vi "udp_test.vi"() -> ()   [LabVIEW 2013]
panel:
  out "data out":string
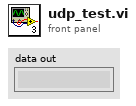
[diagram p1: front panel]
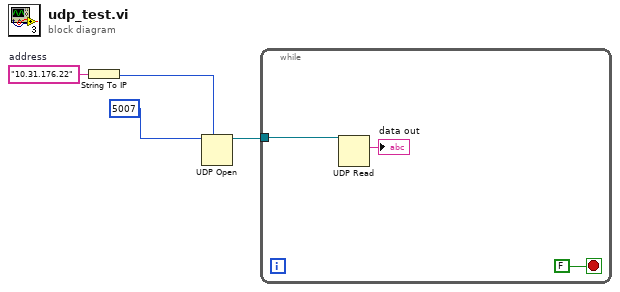
[diagram p0: block diagram]
diagram:
  w4 = "10.31.176.22"  # address
  n1 = String To IP(1:w4) -> (0:w2:u32)
  n2 = UDP Open(7:w2, 11:u16 5007 ("port")) -> (port=w1:refnum<k16>)  [unwired: 3 in, 2 out]
  n3 = while {
    tunnel: w1 -> [w7]
    stop <- FALSE stop-if-true
    n4 = UDP Read(connection ID=w7) -> (data out=→"data out":string)  [unwired: 3 in, 4 out]
  }
